vi "test.vi"(11 "invalue":dbl) -> (3 "characters":dbl)   [LabVIEW 2024]
panel:
  in  "Python path":path
  in  "function name":string
  in  "module path":path
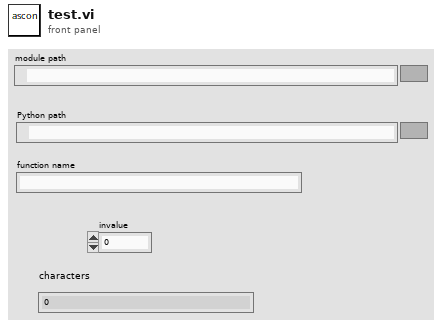
[diagram p1: front panel]
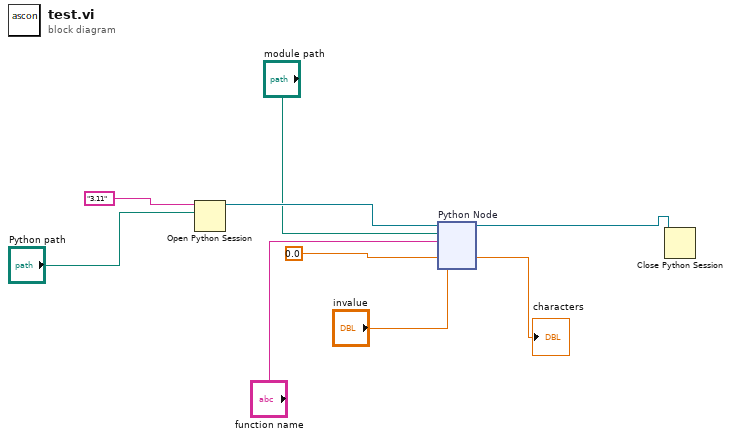
[diagram p0: block diagram]
diagram:
  n1 = Open Python Session(python version="3.11" ("Python version"), python path="Python path") -> (session out=w8:refnum<k35>)  [unwired: 1 in, 1 out]
  n2 = node "Python Node"(w8, "module path", "function name", 0.0, "invalue") -> (w2:refnum<k35>, →"characters":dbl)  [unwired: 2 in, 3 out]
  n3 = Close Python Session(session in=w2) -> ()  [unwired: 1 in, 1 out]
